vi "create_SMGR02.vi"(4 "time_shift":dbl=3.0, 6 "error out in":errorcluster, 7 "array":waveform(i16)[][](array[waveform]), 8 "meas_point":i32, 9 "sync":waveform(i16)) -> (0 "error out":errorcluster, 3 "path":path)   [LabVIEW 2010]
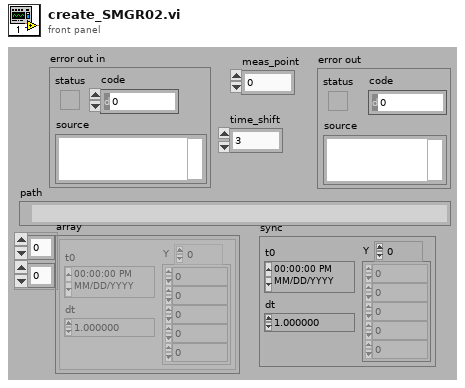
[diagram p1: front panel]
types:
  T1 = enum16{"open", "replace", "create", "open or create", "replace or create", "replace or create with confirmation"}
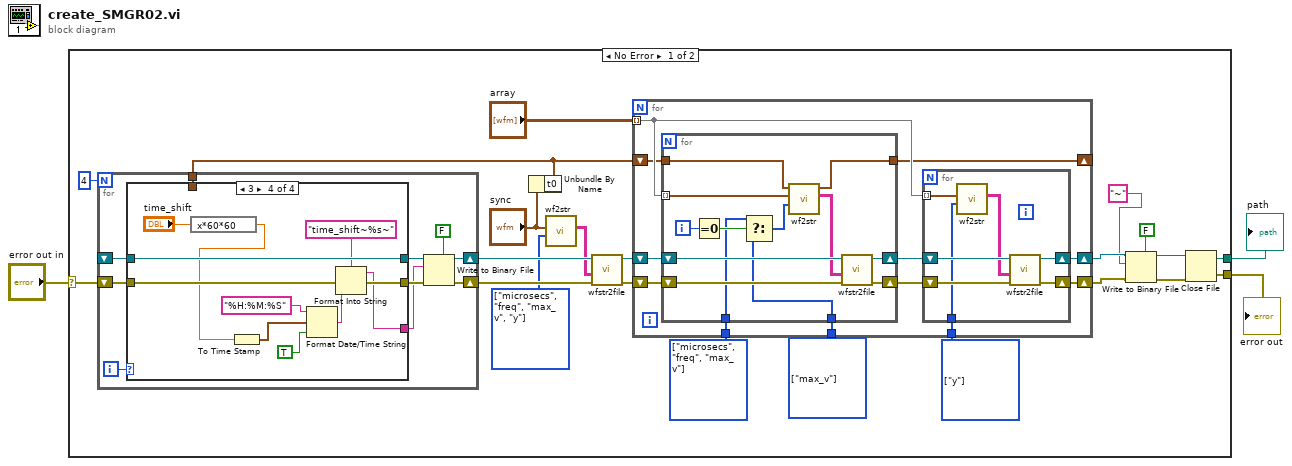
[diagram p0: block diagram]
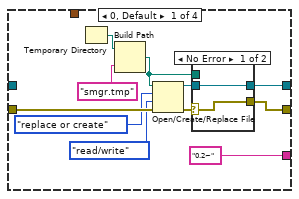
[diagram p2: hidden frame]
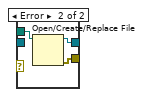
[diagram p3: hidden frame]
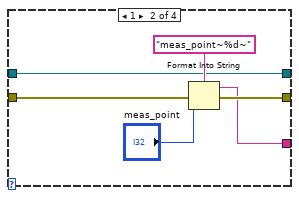
[diagram p4: hidden frame]
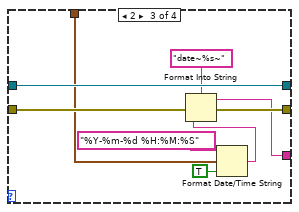
[diagram p5: hidden frame]
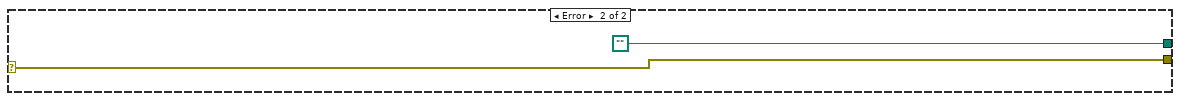
[diagram p6: hidden frame]
diagram:
  n1 = case shown="No Error" "error out in" {
    selector: "error out in" -> [w22 w111]
    tunnel: [w25 w111] -> w2
    tunnel: [w24 path ""] -> w1
    frame No Error {
      w15 = enum16{"microsecs", "freq", "max_v", "y"}[] [enum."y"] items=["microsecs", "freq", "max_v", "y"] ("fields")
      w16 = enum16{"microsecs", "freq", "max_v", "y"}[] [enum."max_v"] items=["microsecs", "freq", "max_v", "y"] ("fields")
      w17 = enum16{"microsecs", "freq", "max_v", "y"}[] [enum."microsecs", enum."freq", enum."max_v"] items=["microsecs", "freq", "max_v", "y"] ("fields")
      w18 = enum16{"microsecs", "freq", "max_v", "y"}[] [enum."microsecs", enum."freq", enum."max_v", enum."y"] items=["microsecs", "freq", "max_v", "y"] ("fields")
      n2 = Unbundle By Name("sync") -> ("t0"=w10:timestamp)
      n3 = for {
        N: 4 -> [_]
        shift-right: [w30] -> w20
        shift-left: _ -> [w33]
        shift-right: [w29] -> w21
        shift-left: w22 -> [w34]
        tunnel: w10 -> [w27]
        i -> [w35]
        n4 = case shown="3" w35 {
          tunnel: [w39 w53 w63 w75] -> w32
          tunnel: [w40 w54 w65 w77] -> w31
          tunnel: w34 -> [w41 w55 w64 w76]
          tunnel: w33 -> [_ w54 w65 w77]
          tunnel: ["0.2~" w52 w60 w70] -> w28
          tunnel: w27 -> [_ _ w59 _]
          frame 0, Default {
            n5 = Temporary Directory() -> (w44:path)
            n6 = Build Path(base path=w44, name or relative path="smgr.tmp") -> (appended path=w42:path)
            n7 = Open/Create/Replace File(file path (use dialog)=w42, error in=w41, operation (0:open)=T1."replace or create", access (0:read/write)=enum16{"read/write", "read-only", "write-only"}."read/write") -> (refnum out=w46:refnum<file>, error out=w45:errorcluster)  [unwired: 2 in, 1 out]
            n8 = case shown="No Error" w45 {
              selector: w45 -> [w48 _]
              tunnel: [w48 w50] -> w39
              tunnel: w46 -> [w47 _]
              tunnel: [w47 w49] -> w40
              tunnel: w42 -> [_ w51]
              frame No Error {
              }
              frame Error {
                n9 = Open/Create/Replace File(file path (use dialog)=w51) -> (refnum out=w49:refnum<file>, error out=w50:errorcluster)  [unwired: 5 in, 1 out]
              }
            }
          }
          frame 1 {
            n10 = Format Into String(format string="meas_point~%d~", error in=w55, "meas_point") -> (resulting string=w52:string, error out=w53:errorcluster)  [unwired: 1 in]
          }
          frame 2 {
            n11 = Format Date/Time String(time format string (%c)="%Y-%m-%d %H:%M:%S", seconds (now)=w59, UTC format=TRUE) -> (date/time string=w62:string)
            n12 = Format Into String(format string="date~%s~", error in=w64, w62) -> (resulting string=w60:string, error out=w63:errorcluster)  [unwired: 1 in]
          }
          frame 3 {
            n13 = expression code="x*60*60"("time_shift") -> (w68:dbl)
            n14 = To Time Stamp(1:w68) -> (0:w69:timestamp)
            n15 = Format Date/Time String(time format string (%c)="%H:%M:%S", seconds (now)=w69, UTC format=TRUE) -> (date/time string=w71:string)
            n16 = Format Into String(format string="time_shift~%s~", error in=w76, w71) -> (resulting string=w70:string, error out=w75:errorcluster)  [unwired: 1 in]
          }
        }
        n17 = Write to Binary File(file (use dialog)=w31, data=w28, error in=w32, 5:FALSE ("prepend array or string size? (T)")) -> (refnum out=w30:refnum<file>, error out=w29:errorcluster)  [unwired: 2 in, 1 out]
      }
      n18 = call "wf2str.vi"("fields"=w18, "Signal"="sync") -> ("Table"=w19:string[][])  [unwired: 3 in, 2 out]
      n19 = call "wfstr2file.vi"("error in"=w21, "Array"=w19, "Byte Stream File Refnum"=w20) -> ("error out"=w13:errorcluster, "Byte Stream File Refnum 2"=w14:refnum<file>)  [unwired: 3 in]
      n20 = for {
        tunnel: "array" -> [w87] mode=indexing
        shift-right: [w81] -> w9
        shift-left: w14 -> [w83]
        shift-right: [w80] -> w8
        shift-left: w13 -> [w82]
        tunnel: w17 -> [w89]
        tunnel: w16 -> [w88]
        tunnel: w15 -> [w86]
        shift-right: [w78] -> _
        shift-left: w10 -> [w79]
        n21 = for {
          tunnel: w87 -> [w99] mode=indexing
          shift-right: [w109] -> w85
          shift-left: w83 -> [w106]
          shift-right: [w108] -> w84
          shift-left: w82 -> [w107]
          tunnel: w89 -> [w102]
          tunnel: w88 -> [w101]
          tunnel: w79 -> [w98]
          tunnel: [w97] -> w78
          i -> [w103]
          n22 = Equal To 0?(x=w103) -> (x = 0?=w104:bool)
          n23 = Select(t=w102, s=w104, f=w101) -> (s? t:f=w100:enum16{"microsecs", "freq", "max_v", "y"}[])
          n24 = call "wf2str.vi"("fields"=w100, "Signal"=w99, "PrevTime"=w98) -> ("Table"=w105:string[][], "NextTime"=w97:timestamp)  [unwired: 2 in, 1 out]
          n25 = call "wfstr2file.vi"("error in"=w107, "Array"=w105, "Byte Stream File Refnum"=w106) -> ("error out"=w108:errorcluster, "Byte Stream File Refnum 2"=w109:refnum<file>)  [unwired: 3 in]
        }
        n26 = for {
          tunnel: w87 -> [w91] mode=indexing
          shift-right: [w96] -> w81
          shift-left: w85 -> [w93]
          shift-right: [w95] -> w80
          shift-left: w84 -> [w94]
          tunnel: w86 -> [w90]
          n27 = call "wf2str.vi"("fields"=w90, "Signal"=w91) -> ("Table"=w92:string[][])  [unwired: 3 in, 2 out]
          n28 = call "wfstr2file.vi"("error in"=w94, "Array"=w92, "Byte Stream File Refnum"=w93) -> ("error out"=w95:errorcluster, "Byte Stream File Refnum 2"=w96:refnum<file>)  [unwired: 3 in]
        }
      }
      n29 = Write to Binary File(file (use dialog)=w9, data="~", error in=w8, 5:FALSE ("prepend array or string size? (T)")) -> (refnum out=w6:refnum<file>, error out=w7:errorcluster)  [unwired: 2 in, 1 out]
      n30 = Close File(refnum=w6, error in=w7) -> (path=w24:path, error out=w25:errorcluster)
    }
    frame Error {
    }
  }
  "error out" <- w2
  "path" <- w1
